vi "Get my IP addresses.vi"(8 "error in (no error)":errorcluster, 11 "Sessions Detected":string[][](array[string])) -> (0 "error out":errorcluster, 3 "Sessions Detected from this PC":string[][](array[string]))   [LabVIEW 2024, in "Session Scanner.lvlib"]
uses:
  Session Scanner.lvlib
  <vilib>/Utility/error.llb/Trim Whitespace One-Sided.vi
panel:
  out "MyPC IPv4 Addresses":string[](array[string])
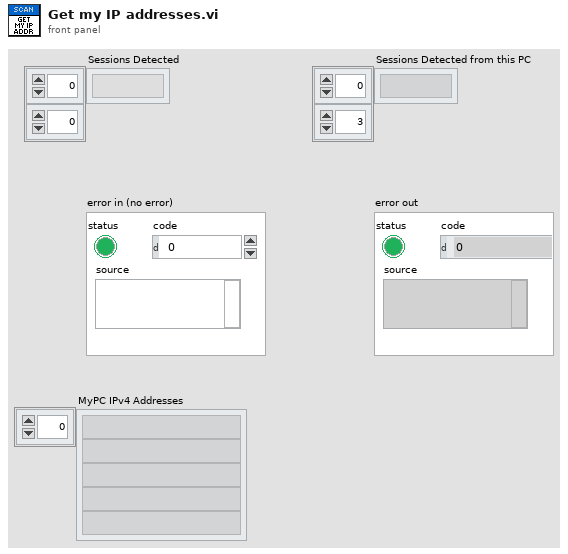
[diagram p1: front panel]
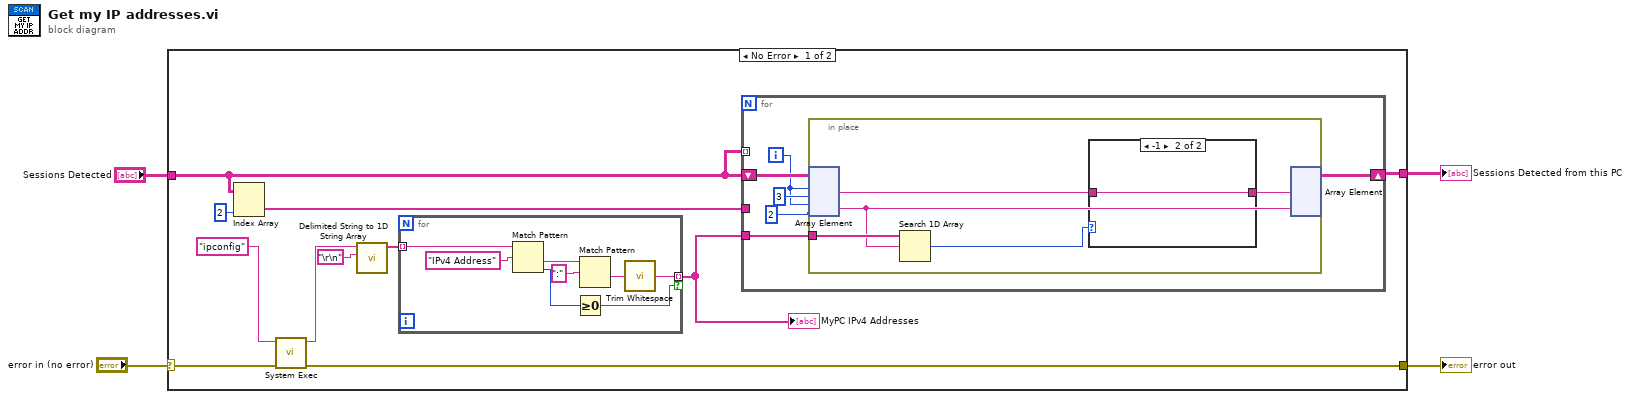
[diagram p0: block diagram]
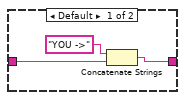
[diagram p2: hidden frame]
diagram:
  n1 = case shown="No Error" "error in (no error)" {
    selector: "error in (no error)" -> [w6 w39]
    tunnel: "Sessions Detected" -> [w5 _]
    tunnel: [w8 _] -> w3
    tunnel: [w7 w39] -> w2
    frame No Error {
      n2 = Index Array(array=w5, index (col)=2) -> (element=w10:string[])  [unwired: 1 in]
      n3 = call <vilib>:"System Exec.vi"("error in (no error)"=w6, "command line"="ipconfig") -> ("error out"=w7:errorcluster, "standard output"=w14:string)  [unwired: 6 in, 2 out]
      n4 = call <vilib>:"Delimited String to 1D String Array.vi"("delimiter"="\r\n", "delimited string"=w14) -> ("string array"=w12:string[])  [unwired: 9 in]
      n5 = for {
        tunnel: w12 -> [w38] mode=indexing
        tunnel: [w31] -> w9 mode=indexing if=w32
        n6 = Match Pattern(string=w38, regular expression="IPv4 Address") -> (after substring=w36:string, offset past match=w33:i32)  [unwired: 1 in, 2 out]
        n7 = Greater Or Equal To 0?(x=w33) -> (x >= 0?=w32:bool)
        n8 = Match Pattern(string=w36, regular expression=":") -> (after substring=w34:string)  [unwired: 1 in, 3 out]
        n9 = call <vilib>:"Trim Whitespace.vi"("string"=w34) -> ("trimmed string"=w31:string)  [unwired: 1 in]
      }
      "MyPC IPv4 Addresses" <- w9
      n10 = for {
        tunnel: w10 -> [_]
        tunnel: w9 -> [w17]
        shift-right: [w16] -> w8
        shift-left: w5 -> [w21]
        tunnel: w5 -> [_] mode=indexing
        i -> [w19]
        n11 = in-place {
          in-place-border: w17 -> [w26]
          n12 = in-place-array #1(w21, w19, 3, w19, 2) -> (w23:string, w25:string)
          n13 = Search 1D Array(1D array=w26, element=w25) -> (index of element=w24:i32)  [unwired: 1 in]
          n14 = case shown="-1" w24 {
            tunnel: w23 -> [w28 w30]
            tunnel: [w27 w30] -> w22
            frame Default {
              n15 = Concatenate Strings("YOU ->" ("string"), w28) -> (w27:string)
            }
            frame -1 {
            }
          }
          n16 = in-place-array #1(w22, w25) -> (w16:string[][])  [unwired: 4 out]
        }
      }
    }
    frame Error {
    }
  }
  "Sessions Detected from this PC" <- w3
  "error out" <- w2
